vi "Configure.vi"(6 "error in":errorcluster, 8 "Configuration":T1, 9 "VISA resource name":refnum<visa-resource-name>) -> (0 "error out":errorcluster, 3 "VISA resource name out":refnum<visa-resource-name>)   [LabVIEW 2023, in "Aim TTi 1908P DMM.lvlib"]
uses:
  Aim TTi 1908P DMM.lvlib
  Configure.ctl
  5ae1b3d7-01ca-4b2a-bb66-f667e26846e6.vi
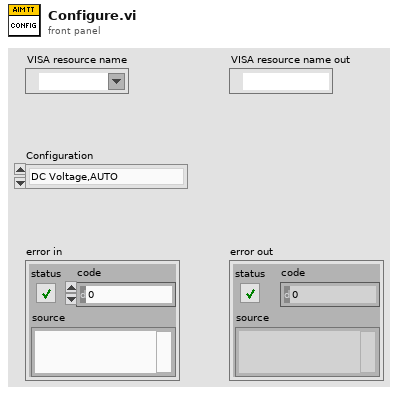
[diagram p1: front panel]
types:
  T1 = typedef "Aim TTi 1908P DMM.lvlib/Configure.ctl" = enum16{"DC Voltage,AUTO", "DC Voltage, 100V", "DC Voltage,10V", "Resistance,AUTO", "Resistance,10K"}
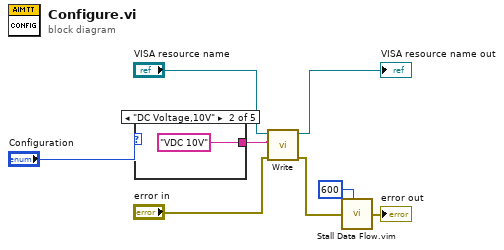
[diagram p0: block diagram]
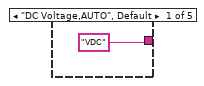
[diagram p2: hidden frame]
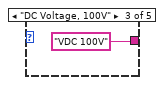
[diagram p3: hidden frame]
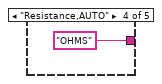
[diagram p4: hidden frame]
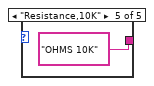
[diagram p5: hidden frame]
diagram:
  n1 = case shown="\"DC Voltage,10V\"" "Configuration" {
    tunnel: ["VDC" ("Data to write") "VDC 10V" ("Data to write") "VDC 100V" ("Data to write") "OHMS" ("Data to write") "OHMS 10K" ("Data to write")] -> w7
    frame "DC Voltage,AUTO", Default {
    }
    frame "DC Voltage,10V" {
    }
    frame "DC Voltage, 100V" {
    }
    frame "Resistance,AUTO" {
    }
    frame "Resistance,10K" {
    }
  }
  n2 = call "Write.vi"("error in"="error in", "Data to write"=w7, "VISA resource name"="VISA resource name") -> ("error out"=w3:errorcluster, "VISA resource name out"=→"VISA resource name out":refnum<visa-resource-name>)  [unwired: 5 in]
  n3 = call "Stall Data Flow.vim"("value in"=w3, "milliseconds to wait"=u32 600) -> ("value out"=→"error out":errorcluster)  [unwired: 1 out]
